vi "整形数值写入.vi"(7 "value":u16, 8 "error in (no error)":errorcluster, 9 "starting address":u16, 10 "Slave ID":u8=1, 11 "MB session in":refnum<class "MB_Master.lvclass">) -> (0 "error out":errorcluster, 3 "MB session out":refnum<class "MB_Master.lvclass">)   [LabVIEW 2016, in "流量计集成.lvlib" / "斯坦道功率测流.lvlib"]
uses:
  <vilib>/Plasmionique/MB Master/MB_Master/MB_Master.lvclass
  <vilib>/Plasmionique/MB Master/MB Master.lvlib
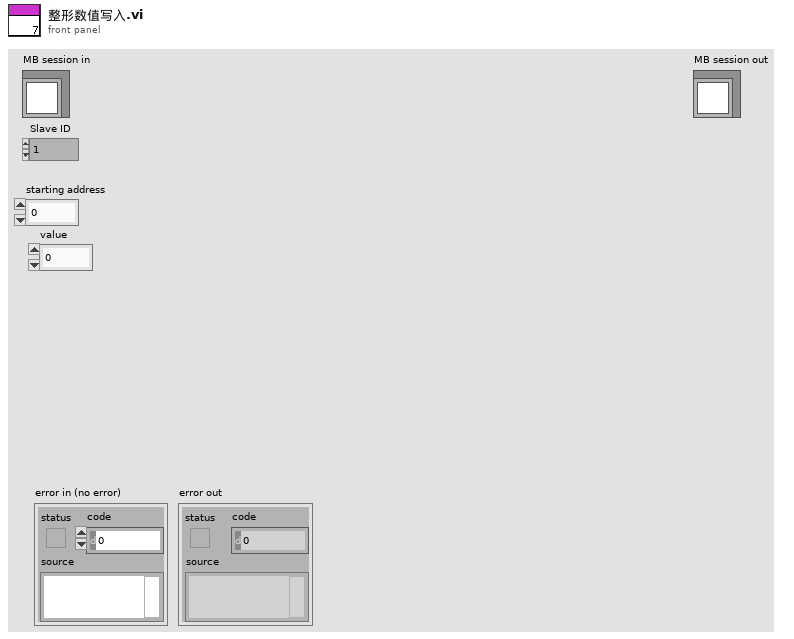
[diagram p1: front panel]
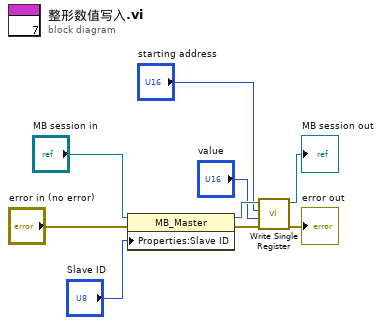
[diagram p0: block diagram]
diagram:
  n1 = property class="MB_Master"(reference="MB session in", error in="error in (no error)", "Properties:Slave ID"="Slave ID") -> (reference out=w6:refnum<class "MB_Master.lvclass">, error out=w4:errorcluster)
  n2 = call <vilib>:"Write Single Register.vi"("error in (no error)"=w4, "value"="value", "address"="starting address", "MB session in"=w6) -> ("error out"=→"error out":errorcluster, "MB session out"=→"MB session out":refnum<class "MB_Master.lvclass">)  [unwired: 6 in]
